vi "lvEtherbone.device_read_single.vi"(0 "eb_socket_ID":i32, 1 "eb_device_ID":i32, 2 "address":u64, 3 "timeout [ms]":i32=1000, 5 "error in (no error)":errorcluster) -> (13 "eb_status":T1, 14 "eb_socket_ID out":i32, 15 "eb_device_ID out":i32, 16 "data":u64, 17 "timed out?":bool, 19 "error out":errorcluster)   [LabVIEW 2009, in "lvEtherbone.lvlib"]
doc: "This is a wrapper around the routine eb_device_read_write. It performs a single Wishbone read cycle."
uses:
  lvEtherbone.lvlib
  lvEtherbone.lveb_status_t.ctl
  lvEtherbone.eb_mode_t.ctl
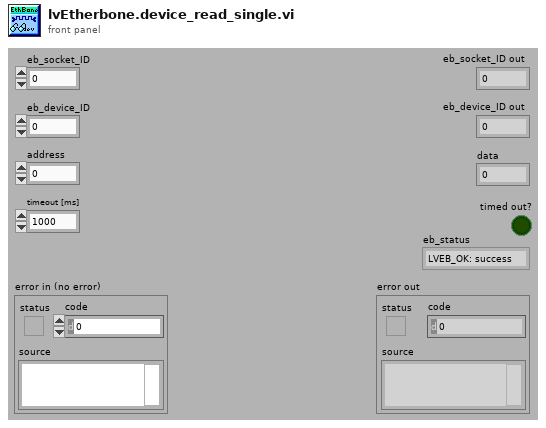
[diagram p1: front panel]
types:
  T1 = typedef "lvEtherbone.lvlib/lvEtherbone.lveb_status_t.ctl" = enum32{"LVEB_OK: success", "LVEB_UNKNOWN: unknown error", "LVEB_OS: operating system forbids access", "LVEB_PORT: port in use or unavailable", "LVEB_ID: ID invalid or out of resources", "LVEB_SOCKET: socket invalid or unavailable", "LVEB_EB: remote address is not Etherbone conformant", "LVEB_IP: bad format or network address", "LVEB_BUSWIDTH: bus width error", "LVEB_DEVICEBUSY: Whishbone device still busy", "LVEB_DEVICEFAIL: operation on Wishbone device failed", "LVEB_DEVICEEXIST: Whishbone device already exists, overlaps, or does not exist", "LVEB_TIMEDOUT: a timeout occurred", "LVEB_OVERFLOW: payload of Etherbone exceeded", "LVEB_ADDRESS: bad address"}
  T2 = typedef "lvEtherbone.lvlib/lvEtherbone.eb_mode_t.ctl" = i32
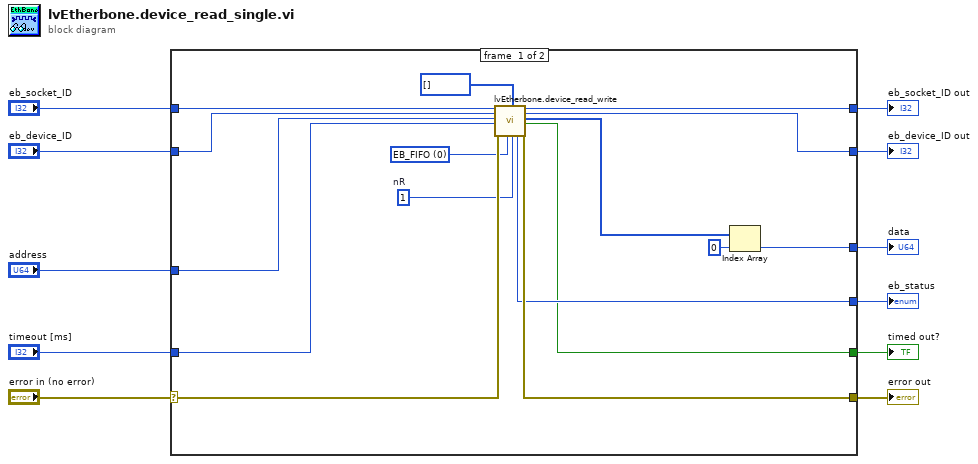
[diagram p0: block diagram]
diagram:
  n1 = case shown="No Error" "error in (no error)" {
    selector: "error in (no error)" -> [w20 w30]
    tunnel: [w19 w30] -> w10
    tunnel: "address" -> [w22 _]
    tunnel: "timeout [ms]" -> [w21 _]
    tunnel: [w15 _] -> w7
    tunnel: [w17 _] -> w6
    tunnel: [w14 _] -> w5
    tunnel: "eb_socket_ID" -> [w27 w29]
    tunnel: [w26 w29] -> w3
    tunnel: "eb_device_ID" -> [w25 w28]
    tunnel: [w24 w28] -> w1
    frame #0 {
      w12 = 1  # nR
      w13 = T2 0 items=["EB_UNDEFINED"=-1, "EB_FIFO"=0, "EB_LINEAR"=1] ("modeR")
      n2 = call "lvEtherbone.device_read_write.vi"("eb_socket_ID"=w27, "eb_device_ID"=w25, "addressR"=w22, "timeout [ms]"=w21, "error in (no error)"=w20, "modeR"=w13, "dataW"=u64[] [], "nR"=w12) -> ("eb_status"=w15:T1, "eb_socket_ID out"=w26:i32, "eb_device_ID out"=w24:i32, "dataR"=w18:u64[], "timed out?"=w14:bool, "error out"=w19:errorcluster)  [unwired: 6 in]
      n3 = Index Array(array=w18, index=0) -> (element=w17:u64)
    }
    frame #1 {
    }
  }
  "error out" <- w10
  "data" <- w6
  "eb_status" <- w7
  "eb_socket_ID out" <- w3
  "eb_device_ID out" <- w1
  "timed out?" <- w5
